vi "Parse General Information.vi"(8 "error in":errorcluster, 11 "VIAnalyzerConfiguration in":refnum<k20>) -> (0 "error out":errorcluster, 2 "StoredCFGPath":path, 3 "VIAnalyzerConfiguration out":refnum<k20>)   [LabVIEW 2020]
uses:
  <vilib>/xml/Close Reference(Node).vi
  <vilib>/xml/NI_XML.lvlib
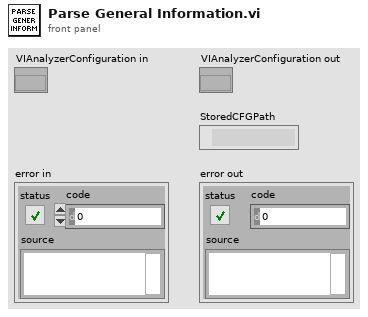
[diagram p1: front panel]
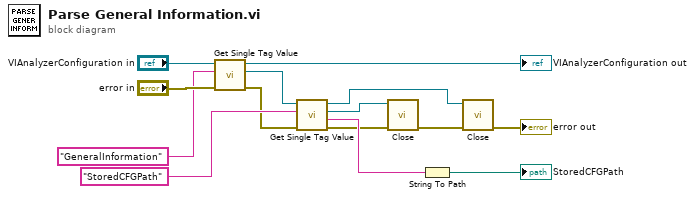
[diagram p0: block diagram]
diagram:
  n1 = call <vilib>:"Get Single Tag Value.vi"("Error In"="error in", "Tag Name"="GeneralInformation", "Element In"="VIAnalyzerConfiguration in") -> ("Error Out"=w6:errorcluster, "Tag Reference"=w7:refnum<k20>, "Element Out"=→"VIAnalyzerConfiguration out":refnum<k20>)  [unwired: 5 in, 1 out]
  n2 = call <vilib>:"Get Single Tag Value.vi"("Error In"=w6, "Tag Name"="StoredCFGPath", "Element In"=w7) -> ("Error Out"=w5:errorcluster, "Tag Value"=w12:string, "Tag Reference"=w4:refnum<k20>, "Element Out"=w2:refnum<k20>)  [unwired: 5 in]
  n3 = call-poly <vilib>:"Close.vi"("error in (no error)"=w5, "node"=w4) -> ("error out"=w3:errorcluster)  [unwired: 7 in]
  n4 = String To Path(string=w12) -> (path=→"StoredCFGPath":path)
  n5 = call-poly <vilib>:"Close.vi"("error in (no error)"=w3, "node"=w2) -> ("error out"=→"error out":errorcluster)  [unwired: 7 in]
